vi "PS directives Generated.vi"(5 "Real In":cluster{"element":fxp<+/-,64,32>, "valid?":bool}, 7 "Imaginary In":cluster{"element":fxp<+/-,64,32>, "valid?":bool}) -> (6 "Power Spectrum":cluster{"element":fxp<+/-,64,32>, "valid?":bool}, 14 "feedback signals":T1)   [LabVIEW 2012]
doc: "This VI is created by the LabVIEW 2012 FPGA IP Builder.\n\nProject: seti_labview.lvproj\nTarget: FPGA Target (PXI-7953R)/IP Builder\nBuild Specification: PS directives\nDirectives Item: PS directives\nTop-Level VI: C:\\work\\seti_fpga\\LabVIEW\\Tester\\PS.vi\n\nEstimated Device Utilization\n-------------------------------------\nSlice Registers: 22.6% (11708 out of 51840)\nSlice LUTs: 28.1% (14578 out of 51840)\nDSP48s: 100.0% (48 out of 48)\nBlock RAMs: 1.6% (3 out of 192)\n\nEstimated Performance\n-------------------------------------\nClock rate (MHz): 250.63\nInitiation interval (cycles): 9750\nPipeline type: Not pipelined\nMinimum latency: 9283\nMaximum latency: 9749"
uses:
  <vilib>/rvi/IPIntegrationNode/IPINode_Utilities/niFpgaIPINodeSimCore.vi
  <vilib>/rvi/IPIntegrationNode/IPINode_Xnode/niFpgaIPINode.xnode
  PS directives Generated Support/IPBlockSimFiles/m3E0CAF06_topH_3F9767D3F620414DAB6EC0B827BFF7CD.dll
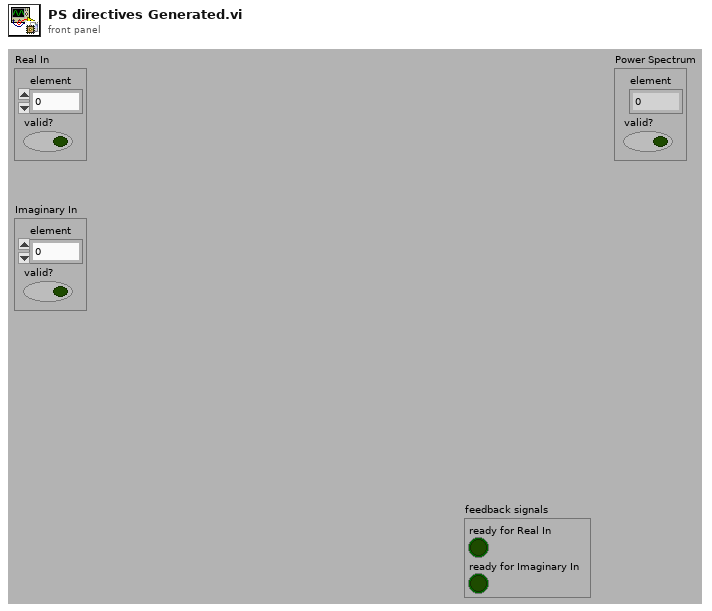
[diagram p1: front panel]
types:
  T1 = cluster{"ready for Real In":bool, "ready for Imaginary In":bool}
  T2 = cluster{"p_Power_Spectrum_2_V_din":fxp<+/-,64,32>, "p_Power_Spectrum_2_vld":bool}
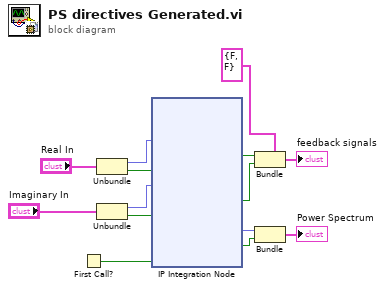
[diagram p0: block diagram]
diagram:
  n1 = First Call?() -> (First Call?: T/F=w14:bool)
  n2 = Unbundle("Real In") -> ("element"=w10:fxp<+/-,64,32>, "valid?"=w9:bool)
  n3 = Unbundle("Imaginary In") -> ("element"=w6:fxp<+/-,64,32>, "valid?"=w5:bool)
  n4 = xnode "IP Integration Node"("p_Real_In_10_V_dout"=w10, "p_Real_In_10_vld"=w9, "p_Imaginary_In_9_V_dout"=w6, "p_Imaginary_In_9_vld"=w5, "first_call"=w14) -> ("ready_for_p_Real_In_10"=w8:bool, "ready_for_p_Imaginary_In_9"=w4:bool, "p_Power_Spectrum_2_V_din"=w2:fxp<+/-,64,32>, "p_Power_Spectrum_2_vld"=w1:bool)  [unwired: 2 in]
  n5 = Bundle ("Bundle_feedback")(cluster=T1 {"ready for Real In"=FALSE, "ready for Imaginary In"=FALSE}, "ready for Real In"=w8, "ready for Imaginary In"=w4) -> (→"feedback signals":T1)
  n6 = Bundle("p_Power_Spectrum_2_V_din"=w2, "p_Power_Spectrum_2_vld"=w1) -> (→"Power Spectrum":T2)  [unwired: 1 in]
